vi "Format CSV.vi"(8 "error in (no error)":errorcluster, 9 "delimiter":string=",", 10 "CSV File Input":path, 11 "Original CSV Format":enum16{"Format A", "Format B"}(ring)) -> (0 "error out":errorcluster, 1 "Parcel Length":i32[](array[numeric]), 2 "All Terminal Data":T1(array[cluster]))   [LabVIEW 2017] (continued)
"24:37.3", "24:37.3", "24:37.4", "24:37.4", "24:37.4", "24:37.5", "24:37.5", "24:37.5", "24:37.6", "24:37.6", "24:37.6", "24:37.7", "24:37.7", "24:37.7", "24:37.8", "24:37.8", "24:37.8", "24:37.9", "24:37.9", "24:37.9", "24:38.0", "24:38.0", "24:38.0", "24:38.1", "24:38.1", "24:38.1", "24:38.2", "24:38.2", "24:38.2", "24:38.3", "24:38.3", "24:38.3", "24:38.4", "24:38.4", "24:38.4", "24:38.5", "24:38.5", "24:38.5", "24:38.6", "24:38.6", "24:38.6", "24:38.7", "24:38.7", "24:38.7", "24:38.8", "24:38.8", "24:38.8", "24:38.9", "24:38.9", "24:38.9", "24:39.0", "24:39.0", "24:39.0", "24:39.1", "24:39.1", "24:39.1", "24:39.2", "24:39.2", "24:39.2", "24:39.3", "24:39.3", "24:39.3", "24:39.4", "24:39.4", "24:39.4", "24:39.5", "24:39.5", "24:39.5", "24:39.6", "24:39.6", "24:39.6", "24:39.7", "24:39.7", "24:39.7", "24:39.8", "24:39.8", "24:39.8", "24:39.9", "24:39.9", "24:39.9", "24:40.0", "24:40.0", "24:40.0", "24:40.1", "24:40.1", "24:40.1", "24:40.2", "24:40.2", "24:40.2", "24:40.3", "24:40.3", "24:40.3", "24:40.4", "24:40.4", "24:40.4", "24:40.5", "24:40.5", "24:40.5", "24:40.6", "24:40.6", "24:40.6", "24:40.7", "24:40.7", "24:40.7", "24:40.8", "24:40.8", "24:40.8", "24:40.9", "24:40.9", "24:40.9", "24:41.0", "24:41.0", "24:41.0", "24:41.1", "24:41.1", "24:41.1", "24:41.2", "24:41.2", "24:41.2", "24:41.3", "24:41.3", "24:41.3", "24:41.4", "24:41.4", "24:41.4", "24:41.5", "24:41.5", "24:41.5", "24:41.6", "24:41.6", "24:41.6", "24:41.7", "24:41.7", "24:41.7", "24:41.8", "24:41.8", "24:41.8", "24:41.9", "24:41.9", "24:41.9", "24:42.0", "24:42.0", "24:42.0", "24:42.1", "24:42.1", "24:42.1", "24:42.2", "24:42.2", "24:42.2", "24:42.3", "24:42.3", "24:42.3", "24:42.4", "24:42.4", "24:42.4", "24:42.5", "24:42.5", "24:42.5", "24:42.6", "24:42.6", "24:42.6", "24:42.7", "24:42.7", "24:42.7", "24:42.8", "24:42.8", "24:42.8", "24:42.9", "24:42.9", "24:42.9", "24:43.0", "24:43.0", "24:43.0", "24:43.1", "24:43.1", "24:43.1", "24:43.2", "24:43.2", "24:43.2", "24:43.3", "24:43.3", "24:43.3", "24:43.4", "24:43.4", "24:43.4", "24:43.5", "24:43.5", "24:43.5", "24:43.6", "24:43.6", "24:43.6", "24:43.7", "24:43.7", "24:43.7", "24:43.8", "24:43.8", "24:43.8", "24:43.9", "24:43.9", "24:43.9", "24:44.0", "24:44.0", "24:44.0", "24:44.1", "24:44.1", "24:44.1", "24:44.2", "24:44.2", "24:44.2", "24:44.3", "24:44.3", "24:44.3", "24:44.4", "24:44.4", "24:44.4", "24:44.5", "24:44.5", "24:44.5", "24:44.6", "24:44.6", "24:44.6", "24:44.7", "24:44.7", "24:44.7", "24:44.8", "24:44.8", "24:44.8", "24:44.9", "24:44.9", "24:44.9", "24:45.0", "24:45.0", "24:45.0", "24:45.1", "24:45.1", "24:45.1", "24:45.2", "24:45.2", "24:45.2", "24:45.3", "24:45.3", "24:45.3", "24:45.4", "24:45.4", "24:45.4", "24:45.5", "24:45.5", "24:45.5", "24:45.6", "24:45.6", "24:45.6", "24:45.7", "24:45.7", "24:45.7", "24:45.8", "24:45.8", "24:45.8", "24:45.9", "24:45.9", "24:45.9", "24:46.0", "24:46.0", "24:46.0", "24:46.1", "24:46.1", "24:46.1", "24:46.2", "24:46.2", "24:46.2", "24:46.3", "24:46.3", "24:46.3", "24:46.4", "24:46.4", "24:46.4", "24:46.5", "24:46.5", "24:46.5", "24:46.6", "24:46.6", "24:46.6", "24:46.7", "24:46.7", "24:46.7", "24:46.8", "24:46.8", "24:46.8", "24:46.9", "24:46.9", "24:46.9", "24:47.0", "24:47.0", "24:47.0", "24:47.1", "24:47.1", "24:47.1", "24:47.2", "24:47.2", "24:47.2", "24:47.3", "24:47.3", "24:47.3", "24:47.4", "24:47.4", "24:47.4", "24:47.5", "24:47.5", "24:47.5", "24:47.6", "24:47.6", "24:47.6", "24:47.7", "24:47.7", "24:47.7", "24:47.8", "24:47.8", "24:47.8", "24:47.9", "24:47.9", "24:47.9", "24:48.0", "24:48.0", "24:48.0", "24:48.1", "24:48.1", "24:48.1", "24:48.2", "24:48.2", "24:48.2", "24:48.3", "24:48.3", "24:48.3", "24:48.4", "24:48.4", "24:48.4", "24:48.5", "24:48.5", "24:48.5", "24:48.6", "24:48.6", "24:48.6", "24:48.7", "24:48.7", "24:48.7", "24:48.8", "24:48.8", "24:48.8", "24:48.9", "24:48.9", "24:48.9", "24:49.0", "24:49.0", "24:49.0", "24:49.1", "24:49.1", "24:49.1", "24:49.2", "24:49.2", "24:49.2", "24:49.3", "24:49.3", "24:49.3", "24:49.4", "24:49.4", "24:49.4", "24:49.5", "24:49.5", "24:49.5", "24:49.6", "24:49.6", "24:49.6", "24:49.7", "24:49.7", "24:49.7", "24:49.8", "24:49.8", "24:49.8", "24:49.9", "24:49.9", "24:49.9", "24:50.0", "24:50.0", "24:50.0", "24:50.1", "24:50.1", "24:50.1", "24:50.2", "24:50.2", "24:50.2", "24:50.3", "24:50.3", "24:50.3", "24:50.4", "24:50.4", "24:50.4", "24:50.5", "24:50.5", "24:50.5", "24:50.6", "24:50.6", "24:50.6", "24:50.7", "24:50.7", "24:50.7", "24:50.8", "24:50.8", "24:50.8", "24:50.9", "24:50.9", "24:50.9", "24:51.0", "24:51.0", "24:51.0", "24:51.1", "24:51.1", "24:51.1", "24:51.2", "24:51.2", "24:51.2", "24:51.3", "24:51.3", "24:51.3", "24:51.4", "24:51.4", "24:51.4", "24:51.5", "24:51.5", "24:51.5", "24:51.6", "24:51.6", "24:51.6", "24:51.7", "24:51.7", "24:51.7", "24:51.8", "24:51.8", "24:51.8", "24:51.9", "24:51.9", "24:51.9", "24:52.0", "24:52.0", "24:52.0", "24:52.1", "24:52.1", "24:52.1", "24:52.2", "24:52.2", "24:52.2", "24:52.3", "24:52.3", "24:52.3", "24:52.4", "24:52.4", "24:52.4", "24:52.5", "24:52.5", "24:52.5", "24:52.6", "24:52.6", "24:52.6", "24:52.7", "24:52.7", "24:52.7", "24:52.8", "24:52.8", "24:52.8", "24:52.9", "24:52.9", "24:52.9", "24:53.0", "24:53.0", "24:53.0", "24:53.1", "24:53.1", "24:53.1", "24:53.2", "24:53.2", "24:53.2", "24:53.3", "24:53.3", "24:53.3", "24:53.4", "24:53.4", "24:53.4", "24:53.5", "24:53.5", "24:53.5", "24:53.6", "24:53.6", "24:53.6", "24:53.7", "24:53.7", "24:53.7", "24:53.8", "24:53.8", "24:53.8", "24:53.9", "24:53.9", "24:53.9", "24:54.0", "24:54.0", "24:54.0", "24:54.1", "24:54.1", "24:54.1", "24:54.2", "24:54.2", "24:54.2", "24:54.3", "24:54.3", "24:54.3", "24:54.4", "24:54.4", "24:54.4", "24:54.5", "24:54.5", "24:54.5", "24:54.6", "24:54.6", "24:54.6", "24:54.7", "24:54.7", "24:54.7", "24:54.8", "24:54.8", "24:54.8", "24:54.9", "24:54.9", "24:54.9", "24:55.0", "24:55.0", "24:55.0", "24:55.1", "24:55.1", "24:55.1", "24:55.2", "24:55.2", "24:55.2", "24:55.3", "24:55.3", "24:55.3", "24:55.4", "24:55.4", "24:55.4", "24:55.5", "24:55.5", "24:55.5", "24:55.6", "24:55.6", "24:55.6", "24:55.7", "24:55.7", "24:55.7", "24:55.8", "24:55.8", "24:55.8", "24:55.9", "24:55.9", "24:55.9", "24:56.0", "24:56.0", "24:56.0", "24:56.1", "24:56.1", "24:56.1", "24:56.2", "24:56.2", "24:56.2", "24:56.3", "24:56.3", "24:56.3", "24:56.4", "24:56.4", "24:56.4", "24:56.5", "24:56.5", "24:56.5", "24:56.6", "24:56.6", "24:56.6", "24:56.7", "24:56.7", "24:56.7", "24:56.8", "24:56.8", "24:56.8", "24:56.9", "24:56.9", "24:56.9", "24:57.0", "24:57.0", "24:57.0", "24:57.1", "24:57.1", "24:57.1", "24:57.2", "24:57.2", "24:57.2", "24:57.3", "24:57.3", "24:57.3", "24:57.4", "24:57.4", "24:57.4", "24:57.5", "24:57.5", "24:57.5", "24:57.6", "24:57.6", "24:57.6", "24:57.7", "24:57.7", "24:57.7", "24:57.8", "24:57.8", "24:57.8", "24:57.9", "24:57.9", "24:57.9", "24:58.0", "24:58.0", "24:58.0", "24:58.1", "24:58.1", "24:58.1", "24:58.2", "24:58.2", "24:58.2", "24:58.3", "24:58.3", "24:58.3", "24:58.4", "24:58.4", "24:58.4", "24:58.5", "24:58.5", "24:58.5", "24:58.6", "24:58.6", "24:58.6", "24:58.7", "24:58.7", "24:58.7", "24:58.8", "24:58.8", "24:58.8", "24:58.9", "24:58.9", "24:58.9", "24:59.0", "24:59.0", "24:59.0", "24:59.1", "24:59.1", "24:59.1", "24:59.2", "24:59.2", "24:59.2", "24:59.3", "24:59.3", "24:59.3", "24:59.4", "24:59.4", "24:59.4", "24:59.5", "24:59.5", "24:59.5", "24:59.6", "24:59.6", "24:59.6", "24:59.7", "24:59.7", "24:59.7", "24:59.8", "24:59.8", "24:59.8", "24:59.9", "24:59.9", "24:59.9", "25:00.0", "25:00.0", "25:00.0", "25:00.1", "25:00.1", "25:00.1", "25:00.2", "25:00.2", "25:00.2", "25:00.3", "25:00.3", "25:00.3", "25:00.4", "25:00.4", "25:00.4", "25:00.5", "25:00.5", "25:00.5", "25:00.6", "25:00.6", "25:00.6", "25:00.7", "25:00.7", "25:00.7", "25:00.8", "25:00.8", "25:00.8", "25:00.9", "25:00.9", "25:00.9", "25:01.0", "25:01.0", "25:01.0", "25:01.1", "25:01.1", "25:01.1", "25:01.2", "25:01.2", "25:01.2", "25:01.3", "25:01.3", "25:01.3", "25:01.4", "25:01.4", "25:01.4", "25:01.5", "25:01.5", "25:01.5", "25:01.6", "25:01.6", "25:01.6", "25:01.7", "25:01.7", "25:01.7", "25:01.8", "25:01.8", "25:01.8", "25:01.9", "25:01.9", "25:01.9", "25:02.0", "25:02.0", "25:02.0", "25:02.1", "25:02.1", "25:02.1", "25:02.2", "25:02.2", "25:02.2", "25:02.3", "25:02.3", "25:02.3", "25:02.4", "25:02.4", "25:02.4", "25:02.5", "25:02.5", "25:02.5", "25:02.6", "25:02.6", "25:02.6", "25:02.7", "25:02.7", "25:02.7", "25:02.8", "25:02.8", "25:02.8", "25:02.9", "25:02.9", "25:02.9", "25:03.0", "25:03.0", "25:03.0", "25:03.1", "25:03.1", "25:03.1", "25:03.2", "25:03.2", "25:03.2", "25:03.3", "25:03.3", "25:03.3", "25:03.4", "25:03.4", "25:03.4", "25:03.5", "25:03.5", "25:03.5", "25:03.6", "25:03.6", "25:03.6", "25:03.7", "25:03.7", "25:03.7", "25:03.8", "25:03.8", "25:03.8", "25:03.9", "25:03.9", "25:03.9", "25:04.0", "25:04.0", "25:04.0", "25:04.1", "25:04.1", "25:04.1", "25:04.2", "25:04.2", "25:04.2", "25:04.3", "25:04.3", "25:04.3", "25:04.4", "25:04.4", "25:04.4", "25:04.5", "25:04.5", "25:04.5", "25:04.6", "25:04.6", "25:04.6", "25:04.7", "25:04.7", "25:04.7", "25:04.8", "25:04.8", "25:04.8", "25:04.9", "25:04.9", "25:04.9", "25:05.0", "25:05.0", "25:05.0", "25:05.1", "25:05.1", "25:05.1", "25:05.2", "25:05.2", "25:05.2", "25:05.3", "25:05.3", "25:05.3", "25:05.4", "25:05.4", "25:05.4", "25:05.5", "25:05.5", "25:05.5", "25:05.6", "25:05.6", "25:05.6", "25:05.7", "25:05.7", "25:05.7", "25:05.8", "25:05.8", "25:05.8", "25:05.9", "25:05.9", "25:05.9", "25:06.0", "25:06.0", "25:06.0", "25:06.1", "25:06.1", "25:06.1", "25:06.2", "25:06.2", "25:06.2", "25:06.3", "25:06.3", "25:06.3", "25:06.4", "25:06.4", "25:06.4", "25:06.5", "25:06.5", "25:06.5", "25:06.6", "25:06.6", "25:06.6", "25:06.7", "25:06.7", "25:06.7", "25:06.8", "25:06.8", "25:06.8", "25:06.9", "25:06.9", "25:06.9", "25:07.0", "25:07.0", "25:07.0", "25:07.1", "25:07.1", "25:07.1", "25:07.2", "25:07.2", "25:07.2", "25:07.3", "25:07.3", "25:07.3", "25:07.4", "25:07.4", "25:07.4", "25:07.5", "25:07.5", "25:07.5", "25:07.6", "25:07.6", "25:07.6", "25:07.7", "25:07.7", "25:07.7", "25:07.8", "25:07.8", "25:07.8", "25:07.9", "25:07.9", "25:07.9", "25:08.0", "25:08.0", "25:08.0", "25:08.1", "25:08.1", "25:08.1", "25:08.2", "25:08.2", "25:08.2", "25:08.3", "25:08.3", "25:08.3", "25:08.4", "25:08.4", "25:08.4", "25:08.5", "25:08.5", "25:08.5", "25:08.6", "25:08.6", "25:08.6", "25:08.7", "25:08.7", "25:08.7", "25:08.8", "25:08.8", "25:08.8", "25:08.9", "25:08.9", "25:08.9", "25:09.0", "25:09.0", "25:09.0", "25:09.1", "25:09.1", "25:09.1", "25:09.2", "25:09.2", "25:09.2", "25:09.3", "25:09.3", "25:09.3", "25:09.4", "25:09.4", "25:09.4", "25:09.5", "25:09.5", "25:09.5", "25:09.6", "25:09.6", "25:09.6", "25:09.7", "25:09.7", "25:09.7", "25:09.8", "25:09.8", "25:09.8", "25:09.9", "25:09.9", "25:09.9", "25:10.0", "25:10.0", "25:10.0", "25:10.1", "25:10.1", "25:10.1", "25:10.2", "25:10.2", "25:10.2", "25:10.3", "25:10.3", "25:10.3", "25:10.4", "25:10.4", "25:10.4", "25:10.5", "25:10.5", "25:10.5", "25:10.6", "25:10.6", "25:10.6", "25:10.7", "25:10.7", "25:10.7", "25:10.8", "25:10.8", "25:10.8", "25:10.9", "25:10.9", "25:10.9", "25:11.0", "25:11.0", "25:11.0", "25:11.1", "25:11.1", "25:11.1", "25:11.2", "25:11.2", "25:11.2", "25:11.3", "25:11.3", "25:11.3", "25:11.4", "25:11.4", "25:11.4", "25:11.5", "25:11.5", "25:11.5", "25:11.6", "25:11.6", "25:11.6", "25:11.7", "25:11.7", "25:11.7", "25:11.8", "25:11.8", "25:11.8", "25:11.9", "25:11.9", "25:11.9", "25:12.0", "25:12.0", "25:12.0", "25:12.1", "25:12.1", "25:12.1", "25:12.2", "25:12.2", "25:12.2", "25:12.3", "25:12.3", "25:12.3", "25:12.4", "25:12.4", "25:12.4", "25:12.5", "25:12.5", "25:12.5", "25:12.6", "25:12.6", "25:12.6", "25:12.7", "25:12.7", "25:12.7", "25:12.8", "25:12.8", "25:12.8", "25:12.9", "25:12.9", "25:12.9", "25:13.0", "25:13.0", "25:13.0", "25:13.1", "25:13.1", "25:13.1", "25:13.2", "25:13.2", "25:13.2", "25:13.3", "25:13.3", "25:13.3", "25:13.4", "25:13.4", "25:13.4", "25:13.5", "25:13.5", "25:13.5", "25:13.6", "25:13.6", "25:13.6", "25:13.7", "25:13.7", "25:13.7", "25:13.8", "25:13.8", "25:13.8", "25:13.9", "25:13.9", "25:13.9", "25:14.0", "25:14.0", "25:14.0", "25:14.1", "25:14.1", "25:14.1", "25:14.2", "25:14.2", "25:14.2", "25:14.3", "25:14.3", "25:14.3", "25:14.4", "25:14.4", "25:14.4", "25:14.5", "25:14.5", "25:14.5", "25:14.6", "25:14.6", "25:14.6", "25:14.7", "25:14.7", "25:14.7", "25:14.8", "25:14.8", "25:14.8", "25:14.9", "25:14.9", "25:14.9", "25:15.0", "25:15.0", "25:15.0", "25:15.1", "25:15.1", "25:15.1", "25:15.2", "25:15.2", "25:15.2", "25:15.3", "25:15.3", "25:15.3", "25:15.4", "25:15.4", "25:15.4", "25:15.5", "25:15.5", "25:15.5", "25:15.6", "25:15.6", "25:15.6", "25:15.7", "25:15.7", "25:15.7", "25:15.8", "25:15.8", "25:15.8", "25:15.9", "25:15.9", "25:15.9", "25:16.0", "25:16.0", "25:16.0", "25:16.1", "25:16.1", "25:16.1", "25:16.2", "25:16.2", "25:16.2", "25:16.3", "25:16.3", "25:16.3", "25:16.4", "25:16.4", "25:16.4", "25:16.5", "25:16.5", "25:16.5", "25:16.6", "25:16.6", "25:16.6", "25:16.7", "25:16.7", "25:16.7", "25:16.8", "25:16.8", "25:16.8", "25:16.9", "25:16.9", "25:16.9", "25:17.0", "25:17.0", "25:17.0", "25:17.1", "25:17.1", "25:17.1", "25:17.2", "25:17.2", "25:17.2", "25:17.3", "25:17.3", "25:17.3", "25:17.4", "25:17.4", "25:17.4", "25:17.5", "25:17.5", "25:17.5", "25:17.6", "25:17.6", "25:17.6", "25:17.7", "25:17.7", "25:17.7", "25:17.8", "25:17.8", "25:17.8", "25:17.9", "25:17.9", "25:17.9", "25:18.0", "25:18.0", "25:18.0", "25:18.1", "25:18.1", "25:18.1", "25:18.2", "25:18.2", "25:18.2", "25:18.3", "25:18.3", "25:18.3", "25:18.4", "25:18.4", "25:18.4", "25:18.5", "25:18.5", "25:18.5", "25:18.6", "25:18.6", "25:18.6", "25:18.7", "25:18.7", "25:18.7", "25:18.8", "25:18.8", "25:18.8", "25:18.9", "25:18.9", "25:18.9", "25:19.0", "25:19.0", "25:19.0", "25:19.1", "25:19.1", "25:19.1", "25:19.2", "25:19.2", "25:19.2", "25:19.3", "25:19.3", "25:19.3", "25:19.4", "25:19.4", "25:19.4", "25:19.5", "25:19.5", "25:19.5", "25:19.6", "25:19.6", "25:19.6", "25:19.7", "25:19.7", "25:19.7", "25:19.8", "25:19.8", "25:19.8", "25:19.9", "25:19.9", "25:19.9", "25:20.0", "25:20.0", "25:20.0", "25:20.1", "25:20.1", "25:20.1", "25:20.2", "25:20.2", "25:20.2", "25:20.3", "25:20.3", "25:20.3", "25:20.4", "25:20.4", "25:20.4", "25:20.5", "25:20.5", "25:20.5", "25:20.6", "25:20.6", "25:20.6", "25:20.7", "25:20.7", "25:20.7", "25:20.8", "25:20.8", "25:20.8", "25:20.9", "25:20.9", "25:20.9", "25:21.0", "25:21.0", "25:21.0", "25:21.1", "25:21.1", "25:21.1", "25:21.2", "25:21.2", "25:21.2", "25:21.3", "25:21.3", "25:21.3", "25:21.4", "25:21.4", "25:21.4", "25:21.5", "25:21.5", "25:21.5", "25:21.6", "25:21.6", "25:21.6", "25:21.7", "25:21.7", "25:21.7", "25:21.8", "25:21.8", "25:21.8", "25:21.9", "25:21.9", "25:21.9", "25:22.0", "25:22.0", "25:22.0", "25:22.1", "25:22.1", "25:22.1", "25:22.2", "25:22.2", "25:22.2", "25:22.3", "25:22.3", "25:22.3", "25:22.4", "25:22.4", "25:22.4", "25:22.5", "25:22.5", "25:22.5", "25:22.6", "25:22.6", "25:22.6", "25:22.7", "25:22.7", "25:22.7", "25:22.8", "25:22.8", "25:22.8", "25:22.9", "25:22.9", "25:22.9", "25:23.0", "25:23.0", "25:23.0", "25:23.1", "25:23.1", "25:23.1", "25:23.2", "25:23.2", "25:23.2", "25:23.3", "25:23.3", "25:23.3", "25:23.4", "25:23.4", "25:23.4", "25:23.5", "25:23.5", "25:23.5", "25:23.6", "25:23.6", "25:23.6", "25:23.7", "25:23.7", "25:23.7", "25:23.8", "25:23.8", "25:23.8", "25:23.9", "25:23.9", "25:23.9", "25:24.0", "25:24.0", "25:24.0", "25:24.1", "25:24.1", "25:24.1", "25:24.2", "25:24.2", "25:24.2", "25:24.3", "25:24.3", "25:24.3", "25:24.4", "25:24.4", "25:24.4", "25:24.5", "25:24.5", "25:24.5", "25:24.6", "25:24.6", "25:24.6", "25:24.7", "25:24.7", "25:24.7", "25:24.8", "25:24.8", "25:24.8", "25:24.9", "25:24.9", "25:24.9", "25:25.0", "25:25.0", "25:25.0", "25:25.1", "25:25.1", "25:25.1", "25:25.2", "25:25.2", "25:25.2", "25:25.3", "25:25.3", "25:25.3", "25:25.4", "25:25.4", "25:25.4", "25:25.5", "25:25.5", "25:25.5", "25:25.6", "25:25.6", "25:25.6", "25:25.7", "25:25.7", "25:25.7", "25:25.8", "25:25.8", "25:25.8", "25:25.9", "25:25.9", "25:25.9", "25:26.0", "25:26.0", "25:26.0", "25:26.1", "25:26.1", "25:26.1", "25:26.2", "25:26.2", "25:26.2", "25:26.3", "25:26.3", "25:26.3", "25:26.4", "25:26.4", "25:26.4", "25:26.5", "25:26.5", "25:26.5", "25:26.6", "25:26.6", "25:26.6", "25:26.7", "25:26.7", "25:26.7", "25:26.8", "25:26.8", "25:26.8", "25:26.9", "25:26.9", "25:26.9", "25:27.0", "25:27.0", "25:27.0", "25:27.1", "25:27.1", "25:27.1", "25:27.2", "25:27.2", "25:27.2", "25:27.3", "25:27.3", "25:27.3", "25:27.4", "25:27.4", "25:27.4", "25:27.5", "25:27.5", "25:27.5", "25:27.6", "25:27.6", "25:27.6", "25:27.7", "25:27.7", "25:27.7", "25:27.8", "25:27.8", "25:27.8", "25:27.9", "25:27.9", "25:27.9", "25:28.0", "25:28.0", "25:28.0", "25:28.1", "25:28.1", "25:28.1", "25:28.2", "25:28.2", "25:28.2", "25:28.3", "25:28.3", "25:28.3", "25:28.4", "25:28.4", "25:28.4", "25:28.5", "25:28.5", "25:28.5", "25:28.6", "25:28.6", "25:28.6", "25:28.7", "25:28.7", "25:28.7", "25:28.8", "25:28.8", "25:28.8", "25:28.9", "25:28.9", "25:28.9", "25:29.0", "25:29.0", "25:29.0", "25:29.1", "25:29.1", "25:29.1", "25:29.2", "25:29.2", "25:29.2", "25:29.3", "25:29.3", "25:29.3", "25:29.4", "25:29.4", "25:29.4", "25:29.5", "25:29.5", "25:29.5", "25:29.6", "25:29.6", "25:29.6", "25:29.7", "25:29.7", "25:29.7", "25:29.8", "25:29.8", "25:29.8", "25:29.9", "25:29.9", "25:29.9", "25:30.0", "25:30.0", "25:30.0", "25:30.1", "25:30.1", "25:30.1", "25:30.2", "25:30.2", "25:30.2", "25:30.3", "25:30.3", "25:30.3", "25:30.4", "25:30.4", "25:30.4", "25:30.5", "25:30.5", "25:30.5", "25:30.6", "25:30.6", "25:30.6", "25:30.7", "25:30.7", "25:30.7", "25:30.8", "25:30.8", "25:30.8", "25:30.9", "25:30.9", "25:30.9", "25:31.0", "25:31.0", "25:31.0", "25:31.1", "25:31.1", "25:31.1", "25:31.2", "25:31.2", "25:31.2", "25:31.3", "25:31.3", "25:31.3", "25:31.4", "25:31.4", "25:31.4", "25:31.5", "25:31.5", "25:31.5", "25:31.6", "25:31.6", "25:31.6", "25:31.7", "25:31.7", "25:31.7", "25:31.8", "25:31.8", "25:31.8", "25:31.9", "25:31.9", "25:31.9", "25:32.0", "25:32.0", "25:32.0", "25:32.1", "25:32.1", "25:32.1", "25:32.2", "25:32.2", "25:32.2", "25:32.3", "25:32.3", "25:32.3", "25:32.4", "25:32.4", "25:32.4", "25:32.5", "25:32.5", "25:32.5", "25:32.6", "25:32.6", "25:32.6", "25:32.7", "25:32.7", "25:32.7", "25:32.8", "25:32.8", "25:32.8", "25:32.9", "25:32.9", "25:32.9", "25:33.0", "25:33.0", "25:33.0", "25:33.1", "25:33.1", "25:33.1", "25:33.2", "25:33.2", "25:33.2", "25:33.3", "25:33.3", "25:33.3", "25:33.4", "25:33.4", "25:33.4", "25:33.5", "25:33.5", "25:33.5", "25:33.6", "25:33.6", "25:33.6", "25:33.7", "25:33.7", "25:33.7", "25:33.8", "25:33.8", "25:33.8", "25:33.9", "25:33.9", "25:33.9", "25:34.0", "25:34.0", "25:34.0", "25:34.1", "25:34.1", "25:34.1", "25:34.2", "25:34.2", "25:34.2", "25:34.3", "25:34.3", "25:34.3", "25:34.4", "25:34.4", "25:34.4", "25:34.5", "25:34.5", "25:34.5", "25:34.6", "25:34.6", "25:34.6", "25:34.7", "25:34.7", "25:34.7", "25:34.8", "25:34.8", "25:34.8", "25:34.9", "25:34.9", "25:34.9", "25:35.0", "25:35.0", "25:35.0", "25:35.1", "25:35.1", "25:35.1", "25:35.2", "25:35.2", "25:35.2", "25:35.3", "25:35.3", "25:35.3", "25:35.4", "25:35.4", "25:35.4", "25:35.5", "25:35.5", "25:35.5", "25:35.6", "25:35.6", "25:35.6", "25:35.7", "25:35.7", "25:35.7", "25:35.8", "25:35.8", "25:35.8", "25:35.9", "25:35.9", "25:35.9", "25:36.0", "25:36.0", "25:36.0", "25:36.1", "25:36.1", "25:36.1", "25:36.2", "25:36.2", "25:36.2", "25:36.3", "25:36.3", "25:36.3", "25:36.4", "25:36.4", "25:36.4", "25:36.5", "25:36.5", "25:36.5", "25:36.6", "25:36.6", "25:36.6", "25:36.7", "25:36.7", "25:36.7", "25:36.8", "25:36.8", "25:36.8", "25:36.9", "25:36.9", "25:36.9", "25:37.0", "25:37.0", "25:37.0", "25:37.1", "25:37.1", "25:37.1", "25:37.2", "25:37.2", "25:37.2", "25:37.3", "25:37.3", "25:37.3", "25:37.4", "25:37.4", "25:37.4", "25:37.5", "25:37.5", "25:37.5", "25:37.6", "25:37.6", "25:37.6", "25:37.7", "25:37.7", "25:37.7", "25:37.8", "25:37.8", "25:37.8", "25:37.9", "25:37.9", "25:37.9", "25:38.0", "25:38.0", "25:38.0", "25:38.1", "25:38.1", "25:38.1", "25:38.2", "25:38.2", "25:38.2", "25:38.3", "25:38.3", "25:38.3", "25:38.4", "25:38.4", "25:38.4", "25:38.5", "25:38.5", "25:38.5", "25:38.6", "25:38.6", "25:38.6", "25:38.7", "25:38.7", "25:38.7", "25:38.8", "25:38.8", "25:38.8", "25:38.9", "25:38.9", "25:38.9", "25:39.0", "25:39.0", "25:39.0", "25:39.1", "25:39.1", "25:39.1", "25:39.2", "25:39.2", "25:39.2", "25:39.3", "25:39.3", "25:39.3", "25:39.4", "25:39.4", "25:39.4", "25:39.5", "25:39.5", "25:39.5", "25:39.6", "25:39.6", "25:39.6", "25:39.7", "25:39.7", "25:39.7", "25:39.8", "25:39.8", "25:39.8", "25:39.9", "25:39.9", "25:39.9", "25:40.0", "25:40.0", "25:40.0", "25:40.1", "25:40.1", "25:40.1", "25:40.2", "25:40.2", "25:40.2", "25:40.3", "25:40.3", "25:40.3", "25:40.4", "25:40.4", "25:40.4", "25:40.5", "25:40.5", "25:40.5", "25:40.6", "25:40.6", "25:40.6", "25:40.7", "25:40.7", "25:40.7", "25:40.8", "25:40.8", "25:40.8", "25:40.9", "25:40.9", "25:40.9", "25:41.0", "25:41.0", "25:41.0", "25:41.1", "25:41.1", "25:41.1", "25:41.2", "25:41.2", "25:41.2", "25:41.3", "25:41.3", "25:41.3", "25:41.4", "25:41.4", "25:41.4", "25:41.5", "25:41.5", "25:41.5", "25:41.6", "25:41.6", "25:41.6", "25:41.7", "25:41.7", "25:41.7", "25:41.8", "25:41.8", "25:41.8", "25:41.9", "25:41.9", "25:41.9", "25:42.0", "25:42.0", "25:42.0", "25:42.1", "25:42.1", "25:42.1", "25:42.2", "25:42.2", "25:42.2", "25:42.3", "25:42.3", "25:42.3", "25:42.4", "25:42.4", "25:42.4", "25:42.5", "25:42.5", "25:42.5", "25:42.6", "25:42.6", "25:42.6", "25:42.7", "25:42.7", "25:42.7", "25:42.8", "25:42.8", "25:42.8", "25:42.9", "25:42.9", "25:42.9", "25:43.0", "25:43.0", "25:43.0", "25:43.1", "25:43.1", "25:43.1", "25:43.2", "25:43.2", "25:43.2", "25:43.3", "25:43.3", "25:43.3", "25:43.4", "25:43.4", "25:43.4", "25:43.5", "25:43.5", "25:43.5", "25:43.6", "25:43.6", "25:43.6", "25:43.7", "25:43.7", "25:43.7", "25:43.8", "25:43.8", "25:43.8", "25:43.9", "25:43.9", "25:43.9", "25:44.0", "25:44.0", "25:44.0", "25:44.1", "25:44.1", "25:44.1", "25:44.2", "25:44.2", "25:44.2", "25:44.3", "25:44.3", "25:44.3", "25:44.4", "25:44.4", "25:44.4", "25:44.5", "25:44.5", "25:44.5", "25:44.6", "25:44.6", "25:44.6", "25:44.7", "25:44.7", "25:44.7", "25:44.8", "25:44.8", "25:44.8", "25:44.9", "25:44.9", "25:44.9", "25:45.0", "25:45.0", "25:45.0", "25:45.1", "25:45.1", "25:45.1", "25:45.2", "25:45.2", "25:45.2", "25:45.3", "25:45.3", "25:45.3", "25:45.4", "25:45.4", "25:45.4", "25:45.5", "25:45.5", "25:45.5", "25:45.6", "25:45.6", "25:45.6", "25:45.7", "25:45.7", "25:45.7", "25:45.8", "25:45.8", "25:45.8", "25:45.9", "25:45.9", "25:45.9", "25:46.0", "25:46.0", "25:46.0", "25:46.1", "25:46.1", "25:46.1", "25:46.2", "25:46.2", "25:46.2", "25:46.3", "25:46.3", "25:46.3", "25:46.4", "25:46.4", "25:46.4", "25:46.5", "25:46.5", "25:46.5", "25:46.6", "25:46.6", "25:46.6", "25:46.7", "25:46.7", "25:46.7", "25:46.8", "25:46.8", "25:46.8", "25:46.9", "25:46.9", "25:46.9", "25:47.0", "25:47.0", "25:47.0", "25:47.1", "25:47.1", "25:47.1", "25:47.2", "25:47.2", "25:47.2", "25:47.3", "25:47.3", "25:47.3", "25:47.4", "25:47.4", "25:47.4", "25:47.5", "25:47.5", "25:47.5", "25:47.6", "25:47.6", "25:47.6", "25:47.7", "25:47.7", "25:47.7", "25:47.8", "25:47.8", "25:47.8", "25:47.9", "25:47.9", "25:47.9", "25:48.0", "25:48.0", "25:48.0", "25:48.1", "25:48.1", "25:48.1", "25:48.2", "25:48.2", "25:48.2", "25:48.3", "25:48.3", "25:48.3", "25:48.4", "25:48.4", "25:48.4", "25:48.5", "25:48.5", "25:48.5", "25:48.6", "25:48.6", "25:48.6", "25:48.7", "25:48.7", "25:48.7", "25:48.8", "25:48.8", "25:48.8", "25:48.9", "25:48.9", "25:48.9", "25:49.0", "25:49.0", "25:49.0", "25:49.1", "25:49.1", "25:49.1", "25:49.2", "25:49.2", "25:49.2", "25:49.3", "25:49.3", "25:49.3", "25:49.4", "25:49.4", "25:49.4", "25:49.5", "25:49.5", "25:49.5", "25:49.6", "25:49.6", "25:49.6", "25:49.7", "25:49.7", "25:49.7", "25:49.8", "25:49.8", "25:49.8", "25:49.9", "25:49.9", "25:49.9", "25:50.0", "25:50.0", "25:50.0", "25:50.1", "25:50.1", "25:50.1", "25:50.2", "25:50.2", "25:50.2", "25:50.3", "25:50.3", "25:50.3", "25:50.4", "25:50.4", "25:50.4", "25:50.5", "25:50.5", "25:50.5", "25:50.6", "25:50.6", "25:50.6", "25:50.7", "25:50.7", "25:50.7", "25:50.8", "25:50.8", "25:50.8", "25:50.9", "25:50.9", "25:50.9", "25:51.0", "25:51.0", "25:51.0", "25:51.1", "25:51.1", "25:51.1", "25:51.2", "25:51.2", "25:51.2", "25:51.3", "25:51.3", "25:51.3", "25:51.4", "25:51.4", "25:51.4", "25:51.5", "25:51.5", "25:51.5", "25:51.6", "25:51.6", "25:51.6", "25:51.7", "25:51.7", "25:51.7", "25:51.8", "25:51.8", "25:51.8", "25:51.9", "25:51.9", "25:51.9", "25:52.0", "25:52.0", "25:52.0", "25:52.1", "25:52.1", "25:52.1", "25:52.2", "25:52.2", "25:52.2", "25:52.3", "25:52.3", "25:52.3", "25:52.4", "25:52.4", "25:52.4", "25:52.5", "25:52.5", "25:52.5", "25:52.6", "25:52.6", "25:52.6", "25:52.7", "25:52.7", "25:52.7", "25:52.8", "25:52.8", "25:52.8", "25:52.9", "25:52.9", "25:52.9", "25:53.0", "25:53.0", "25:53.0", "25:53.1", "25:53.1", "25:53.1", "25:53.2", "25:53.2", "25:53.2", "25:53.3", "25:53.3", "25:53.3", "25:53.4", "25:53.4", "25:53.4", "25:53.5", "25:53.5", "25:53.5", "25:53.6", "25:53.6", "25:53.6", "25:53.7", "25:53.7", "25:53.7", "25:53.8", "25:53.8", "25:53.8", "25:53.9", "25:53.9", "25:53.9", "25:54.0", "25:54.0", "25:54.0", "25:54.1", "25:54.1", "25:54.1", "25:54.2", "25:54.2", "25:54.2", "25:54.3", "25:54.3", "25:54.3", "25:54.4", "25:54.4", "25:54.4", "25:54.5", "25:54.5", "25:54.5", "25:54.6", "25:54.6", "25:54.6", "25:54.7", "25:54.7", "25:54.7", "25:54.8", "25:54.8", "25:54.8", "25:54.9", "25:54.9", "25:54.9", "25:55.0", "25:55.0", "25:55.0", "25:55.1", "25:55.1", "25:55.1", "25:55.2", "25:55.2", "25:55.2", "25:55.3", "25:55.3", "25:55.3", "25:55.4", "25:55.4", "25:55.4", "25:55.5", "25:55.5", "25:55.5", "25:55.6", "25:55.6", "25:55.6", "25:55.7", "25:55.7", "25:55.7", "25:55.8", "25:55.8", "25:55.8", "25:55.9", "25:55.9", "25:55.9", "25:56.0", "25:56.0", "25:56.0", "25:56.1", "25:56.1", "25:56.1", "25:56.2", "25:56.2", "25:56.2", "25:56.3", "25:56.3", "25:56.3", "25:56.4", "25:56.4", "25:56.4", "25:56.5", "25:56.5", "25:56.5", "25:56.6", "25:56.6", "25:56.6", "25:56.7", "25:56.7", "25:56.7", "25:56.8", "25:56.8", "25:56.8", "25:56.9", "25:56.9", "25:56.9", "25:57.0", "25:57.0", "25:57.0", "25:57.1", "25:57.1", "25:57.1", "25:57.2", "25:57.2", "25:57.2", "25:57.3", "25:57.3", "25:57.3", "25:57.4", "25:57.4", "25:57.4", "25:57.5", "25:57.5", "25:57.5", "25:57.6", "25:57.6", "25:57.6", "25:57.7", "25:57.7", "25:57.7", "25:57.8", "25:57.8", "25:57.8", "25:57.9", "25:57.9", "25:57.9", "25:58.0", "25:58.0", "25:58.0", "25:58.1", "25:58.1", "25:58.1", "25:58.2", "25:58.2", "25:58.2", "25:58.3", "25:58.3", "25:58.3", "25:58.4", "25:58.4", "25:58.4", "25:58.5", "25:58.5", "25:58.5", "25:58.6", "25:58.6", "25:58.6", "25:58.7", "25:58.7", "25:58.7", "25:58.8", "25:58.8", "25:58.8", "25:58.9", "25:58.9", "25:58.9", "25:59.0", "25:59.0", "25:59.0", "25:59.1", "25:59.1", "25:59.1", "25:59.2", "25:59.2", "25:59.2", "25:59.3", "25:59.3", "25:59.3", "25:59.4", "25:59.4", "25:59.4", "25:59.5", "25:59.5", "25:59.5", "25:59.6", "25:59.6", "25:59.6", "25:59.7", "25:59.7", "25:59.7", "25:59.8", "25:59.8", "25:59.8", "25:59.9", "25:59.9", "25:59.9", "26:00.0", "26:00.0", "26:00.0", "26:00.1", "26:00.1", "26:00.1", "26:00.2", "26:00.2", "26:00.2", "26:00.3", "26:00.3", "26:00.3", "26:00.4", "26:00.4", "26:00.4", "26:00.5", "26:00.5", "26:00.5", "26:00.6", "26:00.6", "26:00.6", "26:00.7", "26:00.7", "26:00.7", "26:00.8", "26:00.8", "26:00.8", "26:00.9", "26:00.9", "26:00.9", "26:01.0", "26:01.0", "26:01.0", "26:01.1", "26:01.1", "26:01.1", "26:01.2", "26:01.2", "26:01.2", "26:01.3", "26:01.3", "26:01.3", "26:01.4", "26:01.4", "26:01.4", "26:01.5", "26:01.5", "26:01.5", "26:01.6", "26:01.6", "26:01.6", "26:01.7", "26:01.7", "26:01.7", "26:01.8", "26:01.8", "26:01.8", "26:01.9", "26:01.9", "26:01.9", "26:02.0", "26:02.0", "26:02.0", "26:02.1", "26:02.1", "26:02.1", "26:02.2", "26:02.2", "26:02.2", "26:02.3", "26:02.3", "26:02.3", "26:02.4", "26:02.4", "26:02.4", "26:02.5", "26:02.5", "26:02.5", "26:02.6", "26:02.6", "26:02.6", "26:02.7", "26:02.7", "26:02.7", "26:02.8", "26:02.8", "26:02.8", "26:02.9", "26:02.9", "26:02.9", "26:03.0", "26:03.0", "26:03.0", "26:03.1", "26:03.1", "26:03.1", "26:03.2", "26:03.2", "26:03.2", "26:03.3", "26:03.3", "26:03.3", "26:03.4", "26:03.4", "26:03.4", "26:03.5", "26:03.5", "26:03.5", "26:03.6", "26:03.6", "26:03.6", "26:03.7", "26:03.7", "26:03.7", "26:03.8", "26:03.8", "26:03.8", "26:03.9", "26:03.9", "26:03.9", "26:04.0", "26:04.0", "26:04.0", "26:04.1", "26:04.1", "26:04.1", "26:04.2", "26:04.2", "26:04.2", "26:04.3", "26:04.3", "26:04.3", "26:04.4", "26:04.4", "26:04.4", "26:04.5", "26:04.5", "26:04.5", "26:04.6", "26:04.6", "26:04.6", "26:04.7", "26:04.7", "26:04.7", "26:04.8", "26:04.8", "26:04.8", "26:04.9", "26:04.9", "26:04.9", "26:05.0", "26:05.0", "26:05.0", "26:05.1", "26:05.1", "26:05.1", "26:05.2", "26:05.2", "26:05.2", "26:05.3", "26:05.3", "26:05.3", "26:05.4", "26:05.4", "26:05.4", "26:05.5", "26:05.5", "26:05.5", "26:05.6", "26:05.6", "26:05.6", "26:05.7", "26:05.7", "26:05.7", "26:05.8", "26:05.8", "26:05.8", "26:05.9", "26:05.9", "26:05.9", "26:06.0", "26:06.0", "26:06.0", "26:06.1", "26:06.1", "26:06.1", "26:06.2", "26:06.2", "26:06.2", "26:06.3", "26:06.3", "26:06.3", "26:06.4", "26:06.4", "26:06.4", "26:06.5", "26:06.5", "26:06.5", "26:06.6", "26:06.6", "26:06.6", "26:06.7", "26:06.7", "26:06.7", "26:06.8", "26:06.8", "26:06.8", "26:06.9", "26:06.9", "26:06.9", "26:07.0", "26:07.0", "26:07.0", "26:07.1", "26:07.1", "26:07.1", "26:07.2", "26:07.2", "26:07.2", "26:07.3", "26:07.3", "26:07.3", "26:07.4", "26:07.4", "26:07.4", "26:07.5", "26:07.5", "26:07.5", "26:07.6", "26:07.6", "26:07.6", "26:07.7", "26:07.7", "26:07.7", "26:07.8", "26:07.8", "26:07.8", "26:07.9", "26:07.9", "26:07.9", "26:08.0", "26:08.0", "26:08.0", "26:08.1", "26:08.1", "26:08.1", "26:08.2", "26:08.2", "26:08.2", "26:08.3", "26:08.3", "26:08.3", "26:08.4", "26:08.4", "26:08.4", "26:08.5", "26:08.5", "26:08.5", "26:08.6", "26:08.6", "26:08.6", "26:08.7", "26:08.7", "26:08.7", "26:08.8", "26:08.8", "26:08.8", "26:08.9", "26:08.9", "26:08.9", "26:09.0", "26:09.0", "26:09.0", "26:09.1", "26:09.1", "26:09.1", "26:09.2", "26:09.2", "26:09.2", "26:09.3", "26:09.3", "26:09.3", "26:09.4", "26:09.4", "26:09.4", "26:09.5", "26:09.5", "26:09.5", "26:09.6", "26:09.6", "26:09.6", "26:09.7", "26:09.7", "26:09.7", "26:09.8", "26:09.8", "26:09.8", "26:09.9", "26:09.9", "26:09.9", "26:10.0", "26:10.0", "26:10.0", "26:10.1", "26:10.1", "26:10.1", "26:10.2", "26:10.2", "26:10.2", "26:10.3", "26:10.3", "26:10.3", "26:10.4", "26:10.4", "26:10.4", "26:10.5", "26:10.5", "26:10.5", "26:10.6", "26:10.6", "26:10.6", "26:10.7", "26:10.7", "26:10.7", "26:10.8", "26:10.8", "26:10.8", "26:10.9", "26:10.9", "26:10.9", "26:11.0", "26:11.0", "26:11.0", "26:11.1", "26:11.1", "26:11.1", "26:11.2", "26:11.2", "26:11.2", "26:11.3", "26:11.3", "26:11.3", "26:11.4", "26:11.4", "26:11.4", "26:11.5", "26:11.5", "26:11.5", "26:11.6", "26:11.6", "26:11.6", "26:11.7", "26:11.7", "26:11.7", "26:11.8", "26:11.8", "26:11.8", "26:11.9", "26:11.9", "26:11.9", "26:12.0", "26:12.0", "26:12.0", "26:12.1", "26:12.1", "26:12.1", "26:12.2", "26:12.2", "26:12.2", "26:12.3", "26:12.3", "26:12.3", "26:12.4", "26:12.4", "26:12.4", "26:12.5", "26:12.5", "26:12.5", "26:12.6", "26:12.6", "26:12.6", "26:12.7", "26:12.7", "26:12.7", "26:12.8", "26:12.8", "26:12.8", "26:12.9", "26:12.9", "26:12.9", "26:13.0", "26:13.0", "26:13.0", "26:13.1", "26:13.1", "26:13.1", "26:13.2", "26:13.2", "26:13.2", "26:13.3", "26:13.3", "26:13.3", "26:13.4", "26:13.4", "26:13.4", "26:13.5", "26:13.5", "26:13.5", "26:13.6", "26:13.6", "26:13.6", "26:13.7", "26:13.7", "26:13.7", "26:13.8", "26:13.8", "26:13.8", "26:13.9", "26:13.9", "26:13.9", "26:14.0", "26:14.0", "26:14.0", "26:14.1", "26:14.1", "26:14.1", "26:14.2", "26:14.2", "26:14.2", "26:14.3", "26:14.3", "26:14.3", "26:14.4", "26:14.4", "26:14.4", "26:14.5", "26:14.5", "26:14.5", "26:14.6", "26:14.6", "26:14.6", "26:14.7", "26:14.7", "26:14.7", "26:14.8", "26:14.8", "26:14.8", "26:14.9", "26:14.9", "26:14.9", "26:15.0", "26:15.0", "26:15.0", "26:15.1", "26:15.1", "26:15.1", "26:15.2", "26:15.2", "26:15.2", "26:15.3", "26:15.3", "26:15.3", "26:15.4", "26:15.4", "26:15.4", "26:15.5", "26:15.5", "26:15.5", "26:15.6", "26:15.6", "26:15.6", "26:15.7", "26:15.7", "26:15.7", "26:15.8", "26:15.8", "26:15.8", "26:15.9", "26:15.9", "26:15.9", "26:16.0", "26:16.0", "26:16.0", "26:16.1", "26:16.1", "26:16.1", "26:16.2", "26:16.2", "26:16.2", "26:16.3", "26:16.3", "26:16.3", "26:16.4", "26:16.4", "26:16.4", "26:16.5", "26:16.5", "26:16.5", "26:16.6", "26:16.6", "26:16.6", "26:16.7", "26:16.7", "26:16.7", "26:16.8", "26:16.8", "26:16.8", "26:16.9", "26:16.9", "26:16.9", "26:17.0", "26:17.0", "26:17.0", "26:17.1", "26:17.1", "26:17.1", "26:17.2", "26:17.2", "26:17.2", "26:17.3", "26:17.3", "26:17.3", "26:17.4", "26:17.4", "26:17.4", "26:17.5", "26:17.5", "26:17.5", "26:17.6", "26:17.6", "26:17.6", "26:17.7", "26:17.7", "26:17.7", "26:17.8", "26:17.8", "26:17.8", "26:17.9", "26:17.9", "26:17.9", "26:18.0", "26:18.0", "26:18.0", "26:18.1", "26:18.1", "26:18.1", "26:18.2", "26:18.2", "26:18.2", "26:18.3", "26:18.3", "26:18.3", "26:18.4", "26:18.4", "26:18.4", "26:18.5", "26:18.5", "26:18.5", "26:18.6", "26:18.6", "26:18.6", "26:18.7", "26:18.7", "26:18.7", "26:18.8", "26:18.8", "26:18.8", "26:18.9", "26:18.9", "26:18.9", "26:19.0", "26:19.0", "26:19.0", "26:19.1", "26:19.1", "26:19.1", "26:19.2", "26:19.2", "26:19.2", "26:19.3", "26:19.3", "26:19.3", "26:19.4", "26:19.4", "26:19.4", "26:19.5", "26:19.5", "26:19.5", "26:19.6", "26:19.6", "26:19.6", "26:19.7", "26:19.7", "26:19.7", "26:19.8", "26:19.8", "26:19.8", "26:19.9", "26:19.9", "26:19.9", "26:20.0", "26:20.0", "26:20.0", "26:20.1", "26:20.1", "26:20.1", "26:20.2", "26:20.2", "26:20.2", "26:20.3", "26:20.3", "26:20.3", "26:20.4", "26:20.4", "26:20.4", "26:20.5", "26:20.5", "26:20.5", "26:20.6", "26:20.6", "26:20.6", "26:20.7", "26:20.7", "26:20.7", "26:20.8", "26:20.8", "26:20.8", "26:20.9", "26:20.9", "26:20.9", "26:21.0", "26:21.0", "26:21.0", "26:21.1", "26:21.1", "26:21.1", "26:21.2", "26:21.2", "26:21.2", "26:21.3", "26:21.3", "26:21.3", "26:21.4", "26:21.4", "26:21.4", "26:21.5", "26:21.5", "26:21.5", "26:21.6", "26:21.6", "26:21.6", "26:21.7", "26:21.7", "26:21.7", "26:21.8", "26:21.8", "26:21.8", "26:21.9", "26:21.9", "26:21.9", "26:22.0", "26:22.0", "26:22.0", "26:22.1", "26:22.1", "26:22.1", "26:22.2", "26:22.2", "26:22.2", "26:22.3", "26:22.3", "26:22.3", "26:22.4", "26:22.4", "26:22.4", "26:22.5", "26:22.5", "26:22.5", "26:22.6", "26:22.6", "26:22.6", "26:22.7", "26:22.7", "26:22.7", "26:22.8", "26:22.8", "26:22.8", "26:22.9", "26:22.9", "26:22.9", "26:23.0", "26:23.0", "26:23.0", "26:23.1", "26:23.1", "26:23.1", "26:23.2", "26:23.2", "26:23.2", "26:23.3", "26:23.3", "26:23.3", "26:23.4", "26:23.4", "26:23.4", "26:23.5", "26:23.5", "26:23.5", "26:23.6", "26:23.6", "26:23.6", "26:23.7", "26:23.7", "26:23.7", "26:23.8", "26:23.8", "26:23.8", "26:23.9", "26:23.9", "26:23.9", "26:24.0", "26:24.0", "26:24.0", "26:24.1", "26:24.1", "26:24.1", "26:24.2", "26:24.2", "26:24.2", "26:24.3", "26:24.3", "26:24.3", "26:24.4", "26:24.4", "26:24.4", "26:24.5", "26:24.5", "26:24.5", "26:24.6", "26:24.6", "26:24.6", "26:24.7", "26:24.7", "26:24.7", "26:24.8", "26:24.8", "26:24.8", "26:24.9", "26:24.9", "26:24.9", "26:25.0", "26:25.0", "26:25.0", "26:25.1", "26:25.1", "26:25.1", "26:25.2", "26:25.2", "26:25.2", "26:25.3", "26:25.3", "26:25.3", "26:25.4", "26:25.4", "26:25.4", "26:25.5", "26:25.5", "26:25.5", "26:25.6", "26:25.6", "26:25.6", "26:25.7", "26:25.7", "26:25.7", "26:25.8", "26:25.8", "26:25.8", "26:25.9", "26:25.9", "26:25.9", "26:26.0", "26:26.0", "26:26.0", "26:26.1", "26:26.1", "26:26.1", "26:26.2", "26:26.2", "26:26.2", "26:26.3", "26:26.3", "26:26.3", "26:26.4", "26:26.4", "26:26.4", "26:26.5", "26:26.5", "26:26.5", "26:26.6", "26:26.6", "26:26.6", "26:26.7", "26:26.7", "26:26.7", "26:26.8", "26:26.8", "26:26.8", "26:26.9", "26:26.9", "26:26.9", "26:27.0", "26:27.0", "26:27.0", "26:27.1", "26:27.1", "26:27.1", "26:27.2", "26:27.2", "26:27.2", "26:27.3", "26:27.3", "26:27.3", "26:27.4", "26:27.4", "26:27.4", "26:27.5", "26:27.5", "26:27.5", "26:27.6", "26:27.6", "26:27.6", "26:27.7", "26:27.7", "26:27.7", "26:27.8", "26:27.8", "26:27.8", "26:27.9", "26:27.9", "26:27.9", "26:28.0", "26:28.0", "26:28.0", "26:28.1", "26:28.1", "26:28.1", "26:28.2", "26:28.2", "26:28.2", "26:28.3", "26:28.3", "26:28.3", "26:28.4", "26:28.4", "26:28.4", "26:28.5", "26:28.5", "26:28.5", "26:28.6", "26:28.6", "26:28.6", "26:28.7", "26:28.7", "26:28.7", "26:28.8", "26:28.8", "26:28.8", "26:28.9", "26:28.9", "26:28.9", "26:29.0", "26:29.0", "26:29.0", "26:29.1", "26:29.1", "26:29.1", "26:29.2", "26:29.2", "26:29.2", "26:29.3", "26:29.3", "26:29.3", "26:29.4", "26:29.4", "26:29.4", "26:29.5", "26:29.5", "26:29.5", "26:29.6", "26:29.6", "26:29.6", "26:29.7", "26:29.7", "26:29.7", "26:29.8", "26:29.8", "26:29.8", "26:29.9", "26:29.9", "26:29.9", "26:30.0", "26:30.0", "26:30.0", "26:30.1", "26:30.1", "26:30.1", "26:30.2", "26:30.2", "26:30.2", "26:30.3", "26:30.3", "26:30.3", "26:30.4", "26:30.4", "26:30.4", "26:30.5", "26:30.5", "26:30.5", "26:30.6", "26:30.6", "26:30.6", "26:30.7", "26:30.7", "26:30.7", "26:30.8", "26:30.8", "26:30.8", "26:30.9", "26:30.9", "26:30.9", "26:31.0", "26:31.0", "26:31.0", "26:31.1", "26:31.1", "26:31.1", "26:31.2", "26:31.2", "26:31.2", "26:31.3", "26:31.3", "26:31.3", "26:31.4", "26:31.4", "26:31.4", "26:31.5", "26:31.5", "26:31.5", "26:31.6", "26:31.6", "26:31.6", "26:31.7", "26:31.7", "26:31.7", "26:31.8", "26:31.8", "26:31.8", "26:31.9", "26:31.9", "26:31.9", "26:32.0", "26:32.0", "26:32.0", "26:32.1", "26:32.1", "26:32.1", "26:32.2", "26:32.2", "26:32.2", "26:32.3", "26:32.3", "26:32.3", "26:32.4", "26:32.4", "26:32.4", "26:32.5", "26:32.5", "26:32.5", "26:32.6", "26:32.6", "26:32.6", "26:32.7", "26:32.7", "26:32.7", "26:32.8", "26:32.8", "26:32.8", "26:32.9", "26:32.9", "26:32.9", "26:33.0", "26:33.0", "26:33.0", "26:33.1", "26:33.1", "26:33.1", "26:33.2", "26:33.2", "26:33.2", "26:33.3", "26:33.3", "26:33.3", "26:33.4", "26:33.4", "26:33.4", "26:33.5", "26:33.5", "26:33.5", "26:33.6", "26:33.6", "26:33.6", "26:33.7", "26:33.7", "26:33.7", "26:33.8", "26:33.8", "26:33.8", "26:33.9", "26:33.9", "26:33.9", "26:34.0", "26:34.0", "26:34.0", "26:34.1", "26:34.1", "26:34.1", "26:34.2", "26:34.2", "26:34.2", "26:34.3", "26:34.3", "26:34.3", "26:34.4", "26:34.4", "26:34.4", "26:34.5", "26:34.5", "26:34.5", "26:34.6", "26:34.6", "26:34.6", "26:34.7", "26:34.7", "26:34.7", "26:34.8", "26:34.8", "26:34.8", "26:34.9", "26:34.9", "26:34.9", "26:35.0", "26:35.0", "26:35.0", "26:35.1", "26:35.1", "26:35.1", "26:35.2", "26:35.2", "26:35.2", "26:35.3", "26:35.3", "26:35.3", "26:35.4", "26:35.4", "26:35.4", "26:35.5", "26:35.5", "26:35.5", "26:35.6", "26:35.6", "26:35.6", "26:35.7", "26:35.7", "26:35.7", "26:35.8", "26:35.8", "26:35.8", "26:35.9", "26:35.9", "26:35.9", "26:36.0", "26:36.0", "26:36.0", "26:36.1", "26:36.1", "26:36.1", "26:36.2", "26:36.2", "26:36.2", "26:36.3", "26:36.3", "26:36.3", "26:36.4", "26:36.4", "26:36.4", "26:36.5", "26:36.5", "26:36.5", "26:36.6", "26:36.6", "26:36.6", "26:36.7", "26:36.7", "26:36.7", "26:36.8", "26:36.8", "26:36.8", "26:36.9", "26:36.9", "26:36.9", "26:37.0", "26:37.0", "26:37.0", "26:37.1", "26:37.1", "26:37.1", "26:37.2", "26:37.2", "26:37.2", "26:37.3", "26:37.3", "26:37.3", "26:37.4", "26:37.4", "26:37.4", "26:37.5", "26:37.5", "26:37.5", "26:37.6", "26:37.6", "26:37.6", "26:37.7", "26:37.7", "26:37.7", "26:37.8", "26:37.8", "26:37.8", "26:37.9", "26:37.9", "26:37.9", "26:38.0", "26:38.0", "26:38.0", "26:38.1", "26:38.1", "26:38.1", "26:38.2", "26:38.2", "26:38.2", "26:38.3", "26:38.3", "26:38.3", "26:38.4", "26:38.4", "26:38.4", "26:38.5",
